vi "List.vi"() -> (0 "error out":errorcluster, 2 "COM ports":string[](array[string]))   [LabVIEW 2013, in "Thorlabs_SC10.lvlib"]
doc: "list all the possible port on this computer.\nserialNo: port list returned string include serial number and device descriptor, separated by comma\nsize: the length of serialNo\n\n\nCOMMANDLIB_API int List(unsigned char *serialNo, int size);"
uses:
  <instrlib>/Thorlabs_SC10/Thorlabs_SC10.lvlib
  <instrlib>/Thorlabs_SC10/Data/SC10CommandLib_win32.dll
  <instrlib>/Thorlabs_SC10/Data/SC10CommandLib_x64.dll
panel:
  in  "error in (no error)":errorcluster
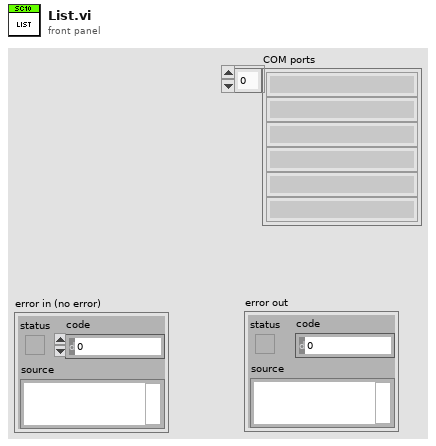
[diagram p1: front panel]
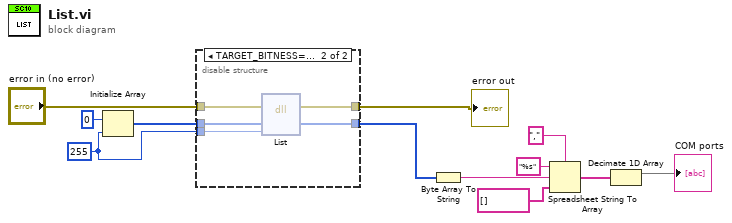
[diagram p0: block diagram]
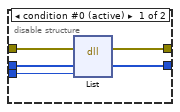
[diagram p2: hidden frame]
diagram:
  w9 = 255 ("dimension size")
  n1 = Initialize Array(u8 0 ("element"), w9) -> (w10:u8[])
  n2 = disable-structure shown="TARGET_BITNESS==64" {
    disable-tunnel: "error in (no error)" -> [w17 w22]
    disable-tunnel: w10 -> [w16 w21]
    disable-tunnel: w9 -> [w15 w20]
    disable-tunnel: [w14 w19] -> w2
    disable-tunnel: [w13 w18] -> w1
    frame condition #0 (active) {
      n3 = dll-call lib="C:/Program Files (x86)/National Instruments/LabVIEW 2013/instr.lib/Thorlabs_SC10/Data/SC10CommandLib_win32.*" fn="List"(error in=w17, "serialNo"=w16, "size"=w15) -> (error out=w14:errorcluster, "serialNo"=w13:u8[])  [unwired: 4 in, 1 out]
    }
    frame condition #1 {
      n4 = dll-call lib="C:/Program Files/National Instruments/LabVIEW 2013/instr.lib/Thorlabs_SC10/Data/SC10CommandLib_x64.dll" fn="List"(error in=w22, "serialNo"=w21, "size"=w20) -> (error out=w19:errorcluster, "serialNo"=w18:u8[])  [unwired: 4 in, 1 out]
    }
  }
  "error out" <- w2
  n5 = Byte Array To String(unsigned byte array=w1) -> (string=w7:string)
  n6 = Spreadsheet String To Array(delimiter (Tab)=",", format string="%s", spreadsheet string=w7, array type (2D Dbl)=string[] []) -> (array=w4:string[])
  n7 = Decimate 1D Array(w4) -> (→"COM ports":string[])  [unwired: 1 out]
